vi "CreateSimulatedData.vi"(8 "error in (no error)":errorcluster) -> (0 "error out":errorcluster, 1 "sampling info":cluster{"Fs":dbl, "#s":dbl}, 2 "simulated tach signal":waveform(sgl), 3 "simulated waveforms":waveform(sgl)[](array[waveform]))   [LabVIEW 2017, in "CmsAcquisition.lvlib"]
uses:
  <vilib>/addons/InsightCM/Devices/Shared/Cms/CmsAcquisition/CmsAcquisition.lvlib
  <vilib>/addons/InsightCM/Devices/Shared/Cms/CmsAcquisition/subVIs/SimulatedConfigRefGlobal.vi
  <vilib>/addons/InsightCM/Utilities/ChannelStatus/ChannelStatus.lvlib
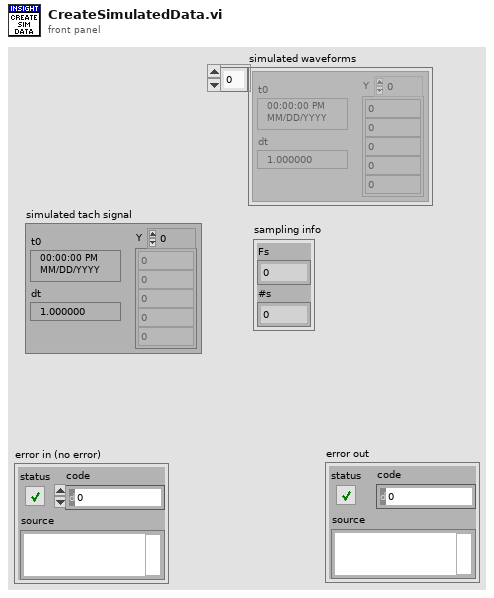
[diagram p1: front panel]
types:
  T1 = typedef "CmsAcquisition.lvlib/AcqSimulated_ConfigRefs.ctl" = cluster{"SignalConfigReference":refnum<vi>, "TachometerConfigReference":refnum<vi>}
  T2 = typedef "FpgaAcquisition923x.lvlib/AcqSimulated_SignalConfig.ctl" = cluster{"SimChannels":T3, "DutyCycle (%)":dbl, "Add Noise?":bool, "NoiseAmplitude":dbl, "Offset":dbl, "SamplingInfo":cluster{"Fs":dbl, "#s":dbl}, "TachMode1-Ch0":bool, "Offsets":dbl[]}
  T3 = typedef "FpgaAcquisition923x.lvlib/AcqSimulated_Channels.ctl" = cluster{"Name":string[], "Vibration":cluster{"order.":dbl, "mag (rms)":dbl, "phase (°)":dbl}[][]}
  T4 = cluster{"order.":dbl, "mag (rms)":dbl, "phase (°)":dbl}[][]
  T5 = cluster{"order.":dbl, "mag (rms)":dbl, "phase (°)":dbl}
  T6 = enum16{"None", "Pk_PkPK", "N Rule", "Z Rule", "U Rule", "Line Noise", "Low Signal", "Ski Slope", "Envelope Test"}
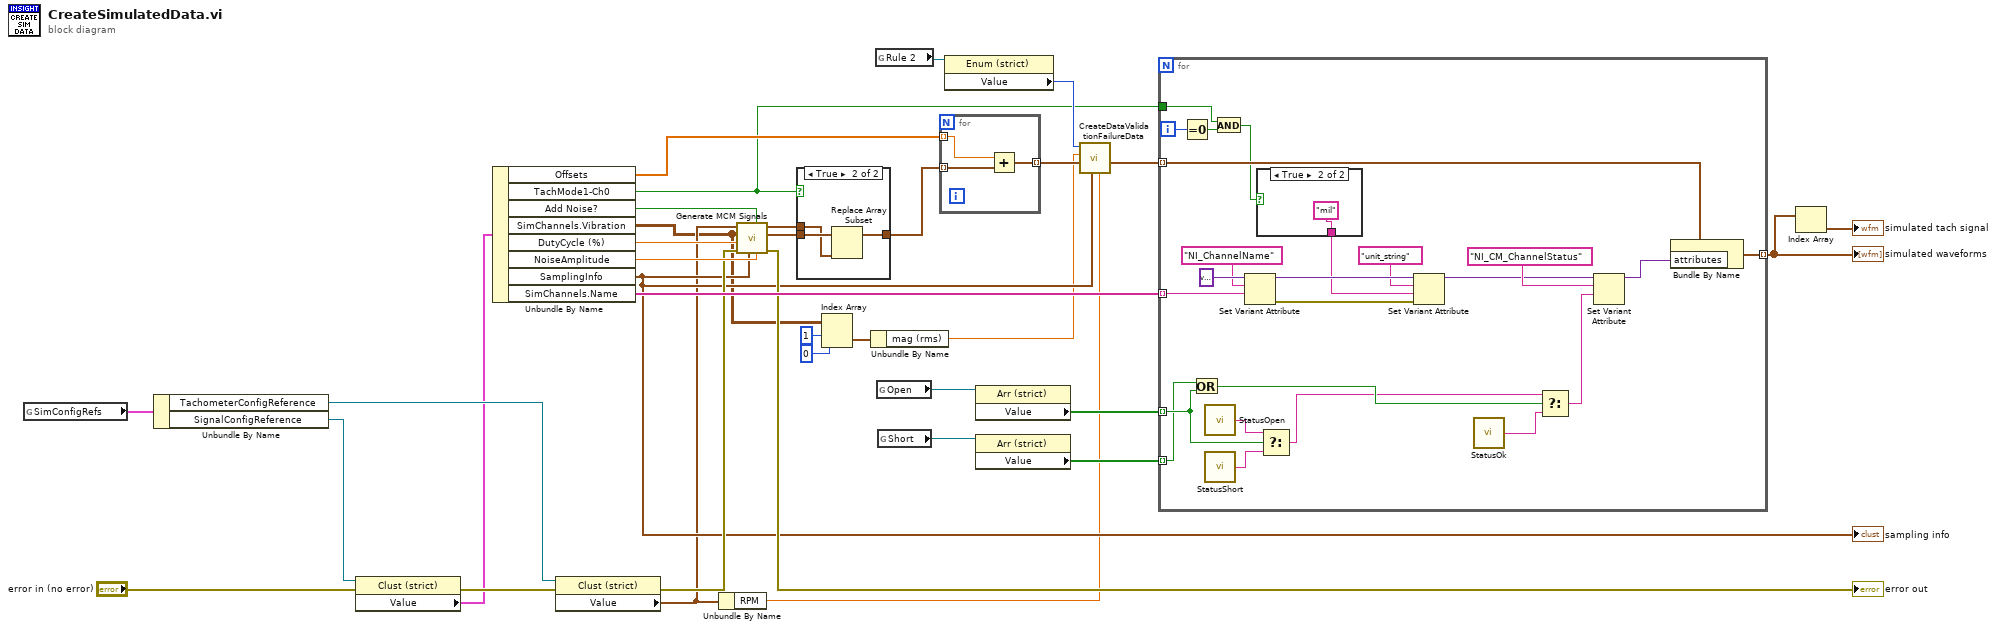
[diagram p0: block diagram]
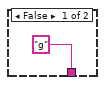
[diagram p3: hidden frame]
diagram:
  n1 = global read "SimulatedConfigRefGlobal.vi" "SimConfigRefs"() -> (w22:T1)
  n2 = Unbundle By Name(w22) -> ("TachometerConfigReference"=w31:refnum<vi>, "SignalConfigReference"=w29:refnum<vi>)
  n3 = property class="Clust (strict)"(reference=w29, error in="error in (no error)") -> (error out=w28:errorcluster, "Value"=w27:T2)  [unwired: 1 out]
  n4 = Unbundle By Name(w27) -> ("Offsets"=w18:dbl[], "TachMode1-Ch0"=w6:bool, "Add Noise?"=w35:bool, "SimChannels.Vibration"=w5:T4, "DutyCycle (%)"=w34:dbl, "NoiseAmplitude"=w33:dbl, "SamplingInfo"=w11:cluster{"Fs":dbl, "#s":dbl}, "SimChannels.Name"=w32:string[])
  "sampling info" <- w11
  n5 = property class="Clust (strict)"(reference=w31, error in=w28) -> (error out=w30:errorcluster, "Value"=w10:cluster{"RPM":sgl})  [unwired: 1 out]
  n6 = Unbundle By Name(w10) -> ("RPM"=w8:sgl)
  n7 = call <vilib>:"Generate MCM Signals.vi"("noise amplitude"=w33, "Add Noise?"=w35, "sampling info"=w11, "error in"=w30, "square wave duty cycle (%)"=w34, "Vibration"=w5, "Tachometer"=w10) -> ("error out"=→"error out":errorcluster, "Vibration signals"=w26:waveform(dbl)[], "Tach signal"=w25:waveform(dbl))  [unwired: 2 in]
  n8 = case shown="True" w6 {
    tunnel: w26 -> [w36 w39]
    tunnel: [w36 w38] -> w19
    tunnel: w25 -> [_ w37]
    frame False {
    }
    frame True {
      n9 = Replace Array Subset(array=w39, new element=w37) -> (w38:waveform(dbl)[])  [unwired: 1 in]
    }
  }
  n10 = Index Array(array=w5, index (row)=1, index (col)=0 ("disabled index (col)")) -> (element=w2:T5)
  n11 = Unbundle By Name(w2) -> ("mag (rms)"=w1:dbl)
  n12 = global read "SimulatedConfigRefGlobal.vi" "Rule 2"() -> (w14:refnum<vi>)
  n13 = global read "SimulatedConfigRefGlobal.vi" "Open"() -> (w17:refnum<vi>)
  n14 = global read "SimulatedConfigRefGlobal.vi" "Short"() -> (w13:refnum<vi>)
  n15 = for {
    tunnel: w19 -> [w42] mode=indexing
    tunnel: w18 -> [w41] mode=indexing
    tunnel: [w40] -> w15 mode=indexing
    n16 = Add(x=w41, y=w42) -> (x+y=w40:waveform(dbl))
  }
  n17 = property class="Enum (strict)"(reference=w14) -> ("Value"=w9:T6)  [unwired: 1 in, 2 out]
  n18 = property class="Arr (strict)"(reference=w17) -> ("Value"=w16:bool[])  [unwired: 1 in, 2 out]
  n19 = property class="Arr (strict)"(reference=w13) -> ("Value"=w12:bool[])  [unwired: 1 in, 2 out]
  n20 = call <vilib>:"CreateDataValidationFailureData.vi"("RPM"=w8, "SamplingInfo"=w11, "in"=w15, "envelope signal amplitude"=w1, "Value 2"=w9) -> ("out"=w7:waveform(dbl)[])  [unwired: 6 in]
  n21 = for {
    tunnel: w7 -> [w61] mode=indexing
    tunnel: [w60] -> w21 mode=indexing
    tunnel: w32 -> [w59] mode=indexing
    tunnel: w16 -> [w51] mode=indexing
    tunnel: w12 -> [w50] mode=indexing
    tunnel: w6 -> [w44]
    i -> [w46]
    n22 = Equal To 0?(x=w46) -> (x = 0?=w45:bool)
    n23 = Or(x=w50, y=w51) -> (x .or. y?=w49:bool)
    n24 = call <vilib>:"StatusOpen.vi"() -> ("status"=w52:string)  [unwired: 5 in]
    n25 = call <vilib>:"StatusShort.vi"() -> ("status"=w53:string)  [unwired: 5 in]
    n26 = And(x=w44, y=w45) -> (x .and. y?=w43:bool)
    n27 = Set Variant Attribute(Variant=variant ("variant out"), name="NI_ChannelName", value=w59) -> (Variant out=w65:variant, error out=w66:errorcluster)  [unwired: 1 in, 1 out]
    n28 = case shown="True" w43 {
      tunnel: ["g" "mil"] -> w58
      frame False {
      }
      frame True {
      }
    }
    n29 = Select(t=w52, s=w51, f=w53) -> (s? t:f=w47:string)
    n30 = Set Variant Attribute(Variant=w65, name="unit_string", value=w58, error in=w66) -> (Variant out=w56:variant)  [unwired: 2 out]
    n31 = call <vilib>:"StatusOk.vi"() -> ("status"=w48:string)  [unwired: 5 in]
    n32 = Select(t=w47, s=w49, f=w48) -> (s? t:f=w54:string)
    n33 = Set Variant Attribute(Variant=w56, name="NI_CM_ChannelStatus", value=w54) -> (Variant out=w55:variant)  [unwired: 1 in, 2 out]
    n34 = Bundle By Name(cluster=w61, "attributes"=w55) -> (w60:waveform(dbl))
  }
  "simulated waveforms" <- w21
  n35 = Index Array(array=w21) -> (element=→"simulated tach signal":waveform(dbl))  [unwired: 1 in]
